vi "BLED1112-Connection retry.vi"(0 "VISA 리소스 이름":refnum<visa-resource-name>="COM8", 5 "MAC Address":string="D3:21:7F:77:05:EF", 7 "Address Type":enum16{"Public", "Random"}(ring)=enum."Random", 11 "에러 입력(에러 없음)":errorcluster) -> (4 "VISA 리소스 이름 출력":refnum<visa-resource-name>="COM8", 6 "Connected":bool=TRUE, 15 "에러 출력":errorcluster={"status"=FALSE, "code"=1073676294, "source"="ble_read_message.vi->ble_read_specific_message.vi->ble_evt_connection_status.vi->BLED1112-Connection retry.vi 안에 VISA 읽기"})   [LabVIEW 2015]
uses:
  Lib_Bled112 toolkit/type_def/connection_status_bundle.ctl
  Lib_Bled112 toolkit/type_def/address_type.ctl
panel:
  out "EVT-bonding":bool=TRUE
  out "Connection Status":T1={"MAC Address"="", "cnx handle"=0, "cnx flags"=0, "Address Type"=125, "Connection Interval (ms)"=125, "Timeout(ms)"=125, "Latency"=0, "bonding handle"=0} {"Address Type" items=["Public", "Random"]}
  out "full message package":u8[](array[numeric])=[0, 3, 6, 3, 0, 0, 0]
  # "BLE connection Retry (w/ Timeout)"
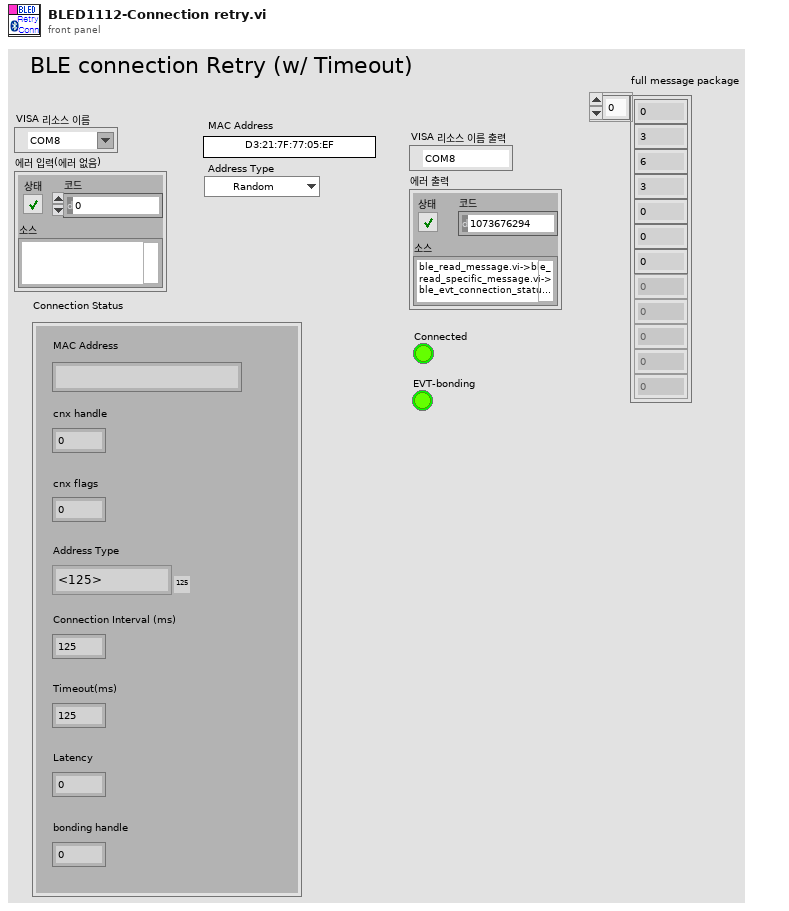
[diagram p1: front panel]
types:
  T1 = typedef "connection_status_bundle.ctl" = cluster{"MAC Address":string, "cnx handle":u8, "cnx flags":u8, "Address Type":T2, "Connection Interval (ms)":u16, "Timeout(ms)":u16, "Latency":u16, "bonding handle":u8}
  T2 = typedef "address_type.ctl" = u8
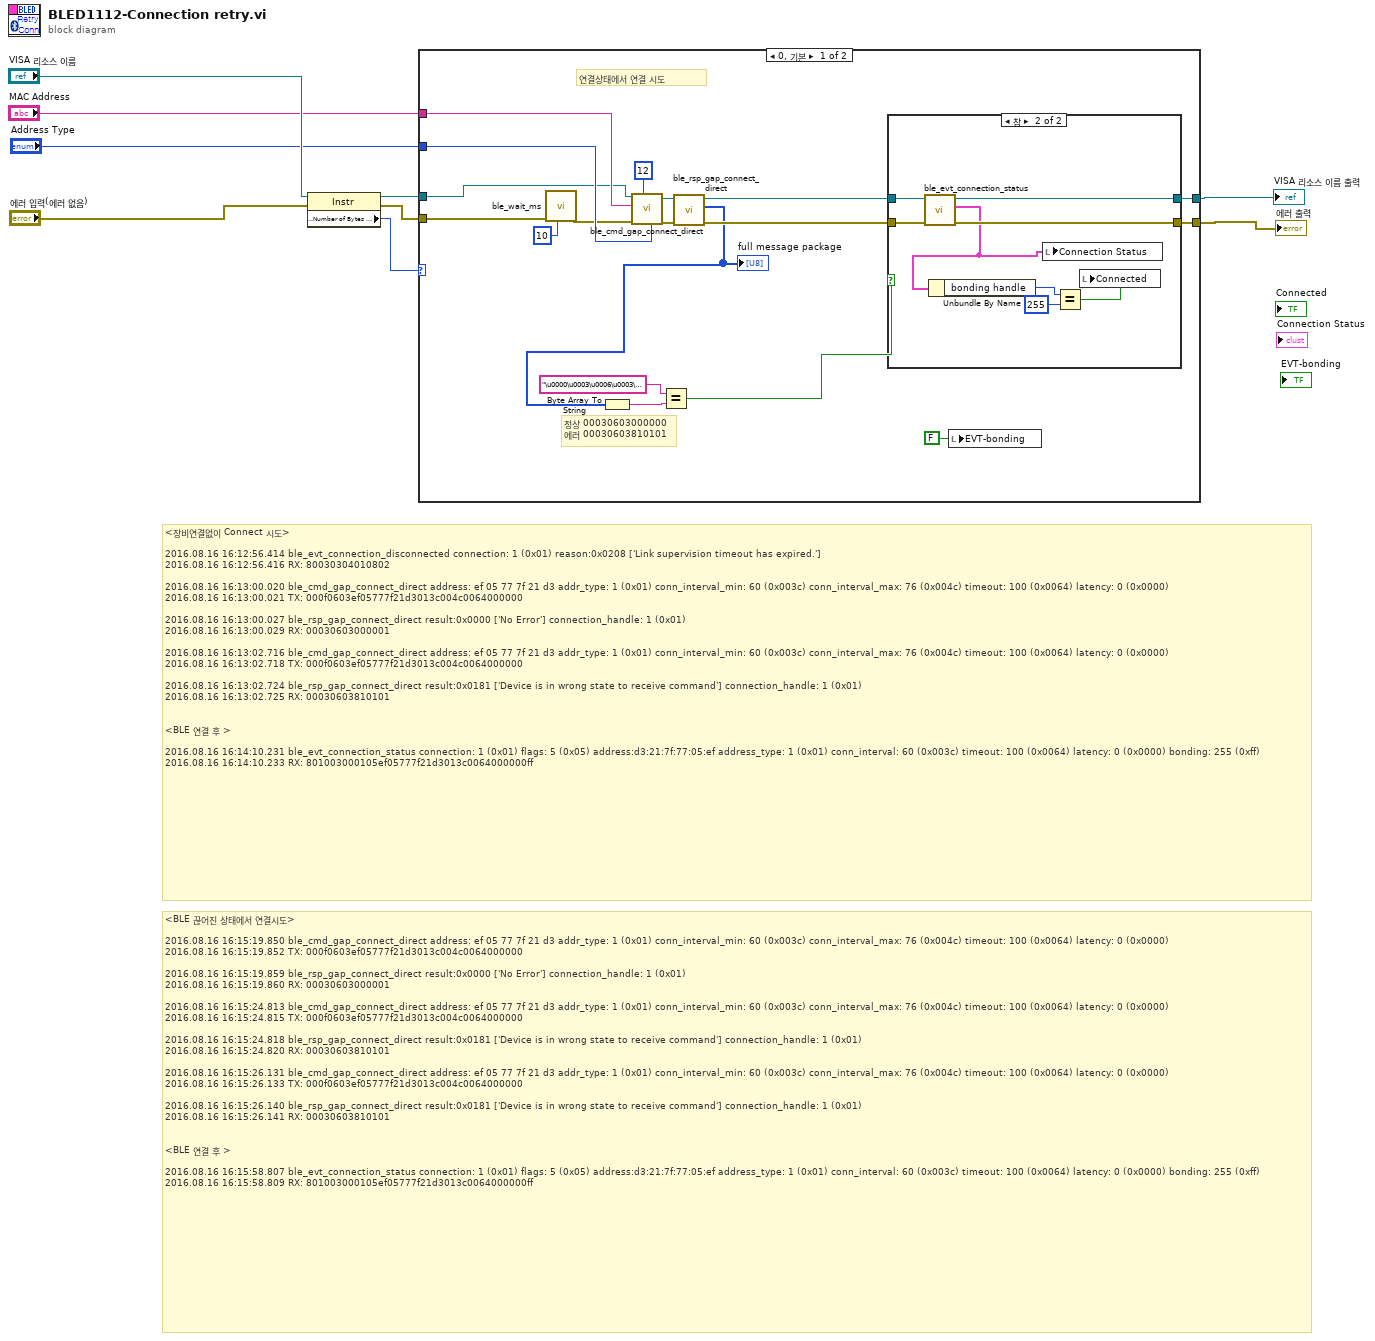
[diagram p0: block diagram]
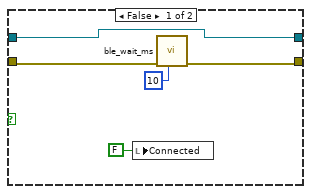
[diagram p2: hidden frame]
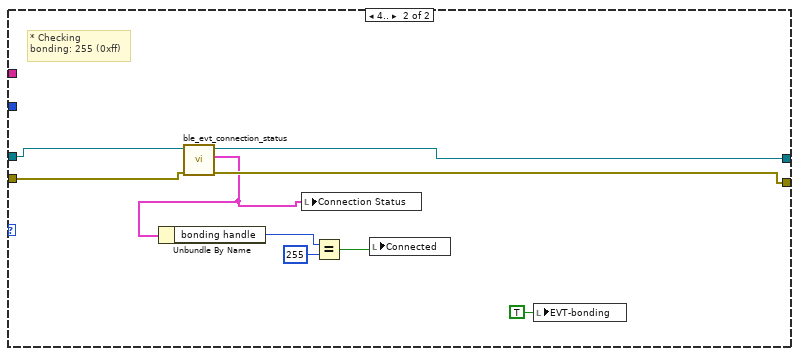
[diagram p3: hidden frame]
diagram:
  # "<BLE 끊어진 상태에서 연결시도>\n\n2016.08.16 16:15:19.850 ble_cmd_gap_connect_direct address: ef 05 77 7f 21 d3 addr_type: 1 (0x01) conn_interval_min: 60 (0x003c) conn_interval_max: 76 (0x004c) timeout: 100 (0x0064) latency: 0 (0x0000)\n2016.08.16 16:15:19.852 TX: 000f0603ef05777f21d3013c004c0064000000\n\n2016.08.16 16:15:19.859 ble_rsp_gap_connect_direct result:0x0000 ['No Error'] connection_handle: 1 (0x01)\n2016.08.16 16:15:19.860 RX: 00030603000001\n\n2016.08.16 16:15:24.813 ble_cmd_gap_connect_direct address: ef 05 77 7f 21 d3 addr_type: 1 (0x01) conn_interval_min: 60 (0x003c) conn_interval_max: 76 (0x004c) timeout: 100 (0x0064) latency: 0 (0x0000)\n2016.08.16 16:15:24.815 TX: 000f0603ef05777f21d3013c004c0064000000\n\n2016.08.16 16:15:24.818 ble_rsp_gap_connect_direct result:0x0181 ['Device is in wrong state to receive command'] connection_handle: 1 (0x01)\n2016.08.16 16:15:24.820 RX: 00030603810101\n\n2016.08.16 16:15:26.131 ble_cmd_gap_connect_direct address: ef 05 77 7f 21 d3 addr_type: 1 (0x01) conn_interval_min: 60 (0x003c) conn_interval_max: 76 (0x004c) timeout: 100 (0x0064) latency: 0 (0x0000)\n2016.08.16 16:15:26.133 TX: 000f0603ef05777f21d3013c004c0064000000\n\n2016.08.16 16:15:26.140 ble_rsp_gap_connect_direct result:0x0181 ['Device is in wrong state to receive command'] connection_handle: 1 (0x01)\n2016.08.16 16:15:26.141 RX: 00030603810101\n\n\n<BLE 연결 후 >\n\n2016.08.16 16:15:58.807 ble_evt_connection_status connection: 1 (0x01) flags: 5 (0x05) address:d3:21:7f:77:05:ef address_type: 1 (0x01) conn_interval: 60 (0x003c) timeout: 100 (0x0064) latency: 0 (0x0000) bonding: 255 (0xff)\n2016.08.16 16:15:58.809 RX: 801003000105ef05777f21d3013c0064000000ff"
  # "<장비연결없이 Connect 시도>\n\n2016.08.16 16:12:56.414 ble_evt_connection_disconnected connection: 1 (0x01) reason:0x0208 ['Link supervision timeout has expired.']\n2016.08.16 16:12:56.416 RX: 80030304010802\n\n2016.08.16 16:13:00.020 ble_cmd_gap_connect_direct address: ef 05 77 7f 21 d3 addr_type: 1 (0x01) conn_interval_min: 60 (0x003c) conn_interval_max: 76 (0x004c) timeout: 100 (0x0064) latency: 0 (0x0000)\n2016.08.16 16:13:00.021 TX: 000f0603ef05777f21d3013c004c0064000000\n\n2016.08.16 16:13:00.027 ble_rsp_gap_connect_direct result:0x0000 ['No Error'] connection_handle: 1 (0x01)\n2016.08.16 16:13:00.029 RX: 00030603000001\n\n2016.08.16 16:13:02.716 ble_cmd_gap_connect_direct address: ef 05 77 7f 21 d3 addr_type: 1 (0x01) conn_interval_min: 60 (0x003c) conn_interval_max: 76 (0x004c) timeout: 100 (0x0064) latency: 0 (0x0000)\n2016.08.16 16:13:02.718 TX: 000f0603ef05777f21d3013c004c0064000000\n\n2016.08.16 16:13:02.724 ble_rsp_gap_connect_direct result:0x0181 ['Device is in wrong state to receive command'] connection_handle: 1 (0x01)\n2016.08.16 16:13:02.725 RX: 00030603810101\n\n\n<BLE 연결 후 >\n\n2016.08.16 16:14:10.231 ble_evt_connection_status connection: 1 (0x01) flags: 5 (0x05) address:d3:21:7f:77:05:ef address_type: 1 (0x01) conn_interval: 60 (0x003c) timeout: 100 (0x0064) latency: 0 (0x0000) bonding: 255 (0xff)\n2016.08.16 16:14:10.233 RX: 801003000105ef05777f21d3013c0064000000ff"
  n1 = property class="Instr"(reference="VISA 리소스 이름", error in="에러 입력(에러 없음)") -> (reference out=w3:refnum<visa-resource-name>, error out=w2:errorcluster, "Serial Settings:Number of Bytes at Serial Port"=w1:u32)
  n2 = case shown="0, 기본" w1 {
    tunnel: "MAC Address" -> [w27 _]
    tunnel: "Address Type" -> [w26 _]
    tunnel: [w15 w45] -> w5
    tunnel: [w14 w44] -> w4
    tunnel: w3 -> [w12 w47]
    tunnel: w2 -> [w11 w46]
    frame 0, Default {
      # "연결상태에서 연결 시도"
      # "정상 00030603000000\n에러 00030603810101"
      n3 = call "ble_wait_ms.vi"("milliseconds to wait (100)"=u32 10, "error in (no error)"=w11) -> ("error out"=w22:errorcluster)  [unwired: 9 in]
      n4 = call "ble_cmd_gap_connect_direct.vi"("Address Type"=w26, "Connection Interval Min (75ms)"=u16 12, "error in (no error)"=w22, "MAC Address"=w27, "COM Bluegiga in"=w12) -> ("error out"=w24:errorcluster, "COM Bluegiga out"=w25:refnum<visa-resource-name>)  [unwired: 5 in]
      n5 = call "ble_rsp_gap_connect_direct.vi"("error in (no error)"=w24, "COM Bluegiga in"=w25) -> ("error out"=w21:errorcluster, "full message package"=w17:u8[], "COM Bluegiga out"=w20:refnum<visa-resource-name>)  [unwired: 7 in]
      "full message package" <- w17
      n6 = Byte Array To String(unsigned byte array=w17) -> (string=w18:string)
      n7 = Equal?(x="\u0000\u0003\u0006\u0003\u0000\u0000\u0000", y=w18) -> (x = y?=w13:bool)
      n8 = case shown="참" w13 {
        tunnel: w21 -> [w31 w40]
        tunnel: w20 -> [w29 w39]
        tunnel: [w29 w38] -> w15
        tunnel: [w30 w37] -> w14
        frame False {
          n9 = local write "Connected"(FALSE ("Connected")) -> ()
          n10 = call "ble_wait_ms.vi"("milliseconds to wait (100)"=u32 10, "error in (no error)"=w31) -> ("error out"=w30:errorcluster)  [unwired: 9 in]
        }
        frame True {
          n11 = call "ble_evt_connection_status.vi"("error in (no error)"=w40, "COM Bluegiga in"=w39) -> ("error out"=w37:errorcluster, "Connection Status"=w33:T1, "COM Bluegiga out"=w38:refnum<visa-resource-name>)  [unwired: 7 in]
          n12 = Unbundle By Name(w33) -> ("bonding handle"=w36:u8)
          n13 = local write "Connection Status"(w33) -> ()
          n14 = Equal?(x=w36, y=u8 255) -> (x = y?=w34:bool)
          n15 = local write "Connected"(w34) -> ()
        }
      }
      n16 = local write "EVT-bonding"(FALSE ("EVT-bonding")) -> ()
    }
    frame 4.. {
      # "* Checking\nbonding: 255 (0xff)"
      n17 = call "ble_evt_connection_status.vi"("error in (no error)"=w46, "COM Bluegiga in"=w47) -> ("error out"=w44:errorcluster, "Connection Status"=w43:T1, "COM Bluegiga out"=w45:refnum<visa-resource-name>)  [unwired: 7 in]
      n18 = Unbundle By Name(w43) -> ("bonding handle"=w49:u8)
      n19 = local write "Connection Status"(w43) -> ()
      n20 = Equal?(x=w49, y=u8 255) -> (x = y?=w42:bool)
      n21 = local write "Connected"(w42) -> ()
      n22 = local write "EVT-bonding"(TRUE ("EVT-bonding")) -> ()
    }
  }
  "VISA 리소스 이름 출력" <- w5
  "에러 출력" <- w4
